vi "List Set Cell Size.vi"(9 "Cell Size":T1={"Width"=27, "Height"=20}, 10 "Cells (N*N)":i32=100, 11 "List Ref In":refnum<vi>) -> (3 "List Ref Out":refnum<vi>)   [LabVIEW 2024]
uses:
  <vilib>/Utility/miscctls.llb/LVBoundsTypeDef.ctl
  <vilib>/Utility/miscctls.llb/LVRowAndColumnTypeDef.ctl
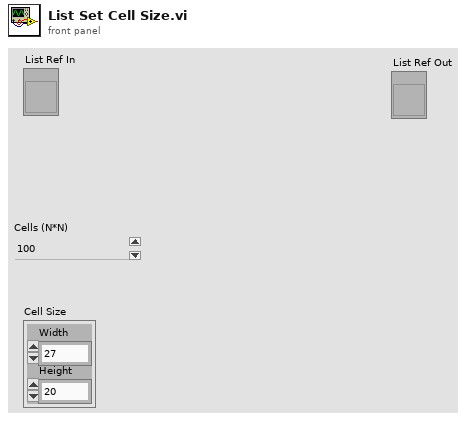
[diagram p1: front panel]
types:
  T1 = typedef "LVBoundsTypeDef.ctl" = cluster{"Width":u32, "Height":u32}
  T2 = typedef "LVRowAndColumnTypeDef.ctl" = cluster{"Row":i32, "Column":i32}
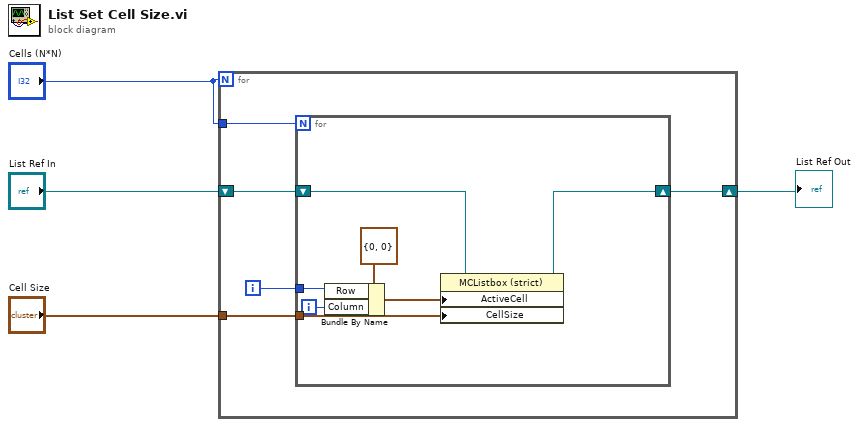
[diagram p0: block diagram]
diagram:
  n1 = for {
    N: "Cells (N*N)" -> [_]
    tunnel: "Cells (N*N)" -> [w8]
    shift-right: [w6] -> w1
    shift-left: "List Ref In" -> [w7]
    tunnel: "Cell Size" -> [w5]
    i -> [w9]
    n2 = for {
      N: w8 -> [_]
      tunnel: w9 -> [w15]
      shift-right: [w11] -> w6
      shift-left: w7 -> [w12]
      tunnel: w5 -> [w10]
      i -> [w14]
      n3 = Bundle By Name(cluster=T2 {"Row"=0, "Column"=0} ("Active Cell:Active Cell"), "Row"=w15, "Column"=w14) -> (w13:T2)
      n4 = property on="Property Node" class="MCListbox (strict)"(reference=w12, "ActiveCell"=w13, "CellSize"=w10) -> (reference out=w11:refnum<vi>)  [unwired: 1 in, 1 out]
    }
  }
  "List Ref Out" <- w1
